vi "FFT Test UI.vi"() -> ()   [LabVIEW 2014]
uses:
  <vilib>/rvi/interface/RandomDataEmulation/nirviRandomDataOpen.vi
  <vilib>/rvi/interface/common/niFpgaCacheSessionInfoDynamic.vi
  <vilib>/rvi/interface/common/niFpgaWaitOnOcc.vi
  <vilib>/Utility/error.llb/Error Cluster From Error Code.vi
  <vilib>/FPGAPlugInAG/Dynamic/niLvFpga_Run_Dynamic.vi
  <vilib>/rvi/errors/niLvFpgaAdjustHostInterfaceError.vi
  <vilib>/FPGAPlugInAG/Dynamic/niLvFpga_Close_Dynamic.vi
  <vilib>/rvi/interface/nirviOpenFPGA/nirviOpenFPGA.xnode
  FFT Test.vi
  <vilib>/rvi/interface/nirviMethod/nirviMethod.xnode
  <vilib>/rvi/interface/nirviCloseFPGA/nirviCloseFPGA.xnode
  <vilib>/FPGAPlugInAG/Dynamic/niLvFpga_ConfigureFifo_Dynamic.vi
  <vilib>/rvi/errors/niLvFpgaMergeErrorWithErrorCode.vi
  <vilib>/FPGAPlugInAG/Dynamic/niLvFpga_StartFifo_Dynamic.vi
  <vilib>/FPGAPlugInAG/Dynamic/niLvFpga_ReadFifo_Dynamic.vi
panel:
  out "FFT Spectrum":waveform(dbl)(graph)={"t0"=timestamp(0 s since 1904-01-01), "dt"=2e-05, "Y"=[]}
  out "Signal":waveform(dbl)(graph)={"t0"=timestamp(0 s since 1904-01-01), "dt"=2e-05, "Y"=[]}
  in  "Stop":bool
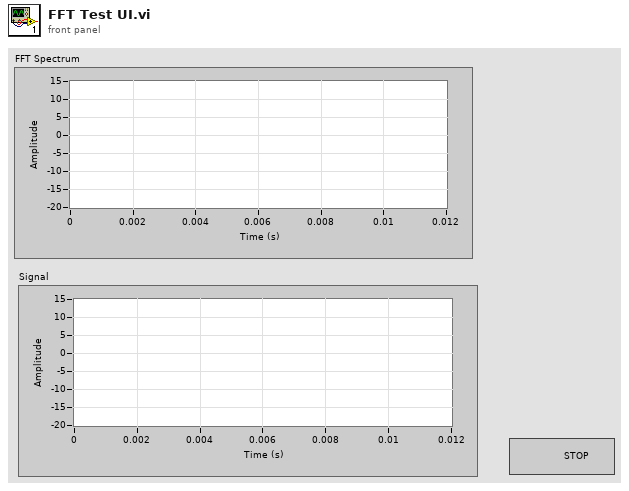
[diagram p1: front panel]
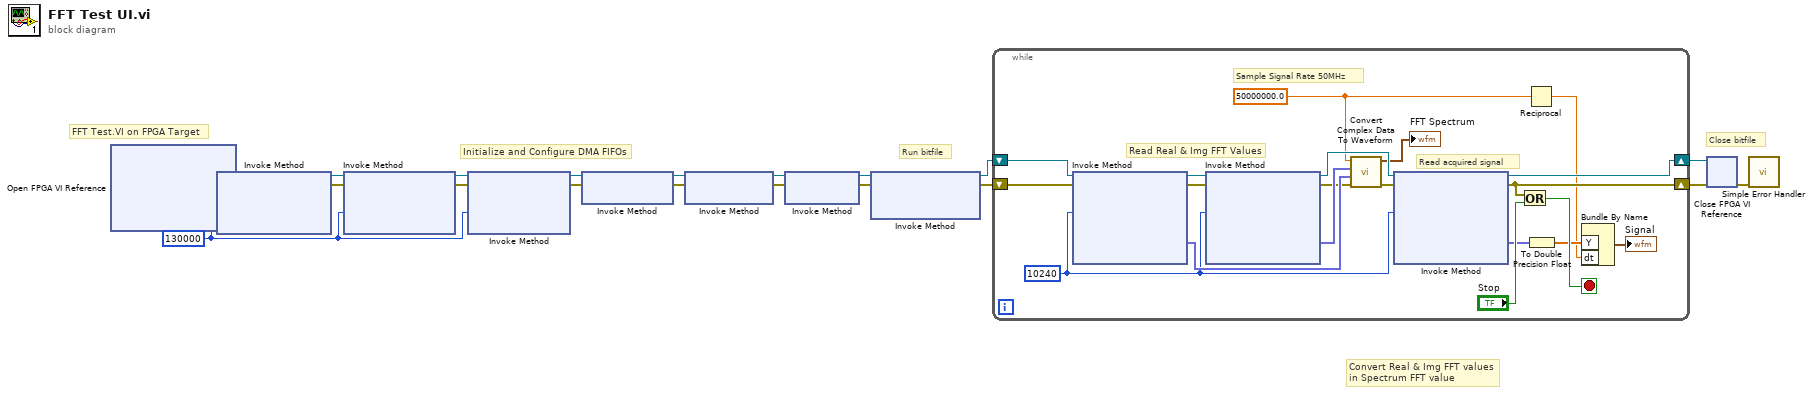
[diagram p0: block diagram]
diagram:
  w8 = u32 130000
  # "FFT Test.VI on FPGA Target"
  # "Close bitfile"
  # "Convert Real & Img FFT values\nin Spectrum FFT value"
  # "Run bitfile"
  # "Initialize and Configure DMA FIFOs"
  n1 = xnode "Open FPGA VI Reference"() -> ("FPGA VI Reference Out"=w7:refnum<k20>, "error out"=w6:errorcluster)  [unwired: 2 in]
  n2 = xnode "Invoke Method"("FPGA VI Reference In"=w7, "error in"=w6, "Requested Depth"=w8) -> ("FPGA VI Reference Out"=w12:refnum<k20>, "error out"=w10:errorcluster)  [unwired: 1 out]
  n3 = xnode "Invoke Method"("FPGA VI Reference In"=w12, "error in"=w10, "Requested Depth"=w8) -> ("FPGA VI Reference Out"=w11:refnum<k20>, "error out"=w9:errorcluster)  [unwired: 1 out]
  n4 = xnode "Invoke Method"("FPGA VI Reference In"=w11, "error in"=w9, "Requested Depth"=w8) -> ("FPGA VI Reference Out"=w19:refnum<k20>, "error out"=w20:errorcluster)  [unwired: 1 out]
  n5 = xnode "Invoke Method"("FPGA VI Reference In"=w19, "error in"=w20) -> ("FPGA VI Reference Out"=w17:refnum<k20>, "error out"=w15:errorcluster)
  n6 = xnode "Invoke Method"("FPGA VI Reference In"=w17, "error in"=w15) -> ("FPGA VI Reference Out"=w18:refnum<k20>, "error out"=w16:errorcluster)
  n7 = xnode "Invoke Method"("FPGA VI Reference In"=w18, "error in"=w16) -> ("FPGA VI Reference Out"=w14:refnum<k20>, "error out"=w13:errorcluster)
  n8 = xnode "Invoke Method"("FPGA VI Reference In"=w14, "error in"=w13) -> ("FPGA VI Reference Out"=w5:refnum<k20>, "error out"=w4:errorcluster)  [unwired: 1 in]
  n9 = while {
    shift-right: [w30] -> w1
    shift-left: w5 -> [w40]
    shift-right: [w28] -> w2
    shift-left: w4 -> [w39]
    stop <- w27 stop-if-true
    w23 = 50000000.0 ("Sample Rate (S/s)")
    w31 = u32 10240 ("Number of Elements")
    # "Read acquired signal"
    # "Read Real & Img FFT Values"
    # "Sample Signal Rate 50MHz"
    n10 = xnode "Invoke Method"("FPGA VI Reference In"=w40, "error in"=w39, "Number of Elements"=w31) -> ("FPGA VI Reference Out"=w38:refnum<k20>, "error out"=w37:errorcluster, "Data"=w35:fxp<+/-,21,14>[])  [unwired: 1 in, 1 out]
    n11 = xnode "Invoke Method"("FPGA VI Reference In"=w38, "error in"=w37, "Number of Elements"=w31) -> ("FPGA VI Reference Out"=w32:refnum<k20>, "error out"=w34:errorcluster, "Data"=w36:fxp<+/-,21,14>[])  [unwired: 1 in, 1 out]
    n12 = call "Convert Complex Data To Waveform.vi"("error in"=w34, "Real Data"=w35, "Imaginary Data"=w36, "Sample Rate (S/s)"=w23) -> ("error out"=w33:errorcluster, "Waveform"=→"FFT Spectrum":waveform(dbl))  [unwired: 6 in]
    n13 = xnode "Invoke Method"("FPGA VI Reference In"=w32, "error in"=w33, "Number of Elements"=w31) -> ("FPGA VI Reference Out"=w30:refnum<k20>, "error out"=w28:errorcluster, "Data"=w26:fxp<+/-,12,5>[])  [unwired: 1 in, 1 out]
    n14 = Or(x=w28, y="Stop") -> (x .or. y?=w27:bool)
    n15 = Reciprocal(x=w23) -> (1/x=w22:dbl)
    n16 = To Double Precision Float(number=w26) -> (double precision float=w24:dbl[])
    n17 = Bundle By Name("Y"=w24, "dt"=w22) -> (→"Signal":waveform(dbl))  [unwired: 1 in]
  }
  n18 = xnode "Close FPGA VI Reference"("FPGA VI Reference In"=w1, "error in"=w2) -> ("error out"=w3:errorcluster)
  n19 = call <vilib>:"Simple Error Handler.vi"("error in (no error)"=w3) -> ()  [unwired: 4 in, 5 out]
